vi "Spectrogram demo.vi"() -> ()   [LabVIEW 2018]
uses:
  <vilib>/Analysis/NI_AALBase.lvlib
  <vilib>/gmath/NI_Gmath.lvlib
  <vilib>/Analysis/NI_AALPro.lvlib
panel:
  in  "Stop":bool
  out "STFT Spectrogram":dbl[][](graph)
  in  "Signal":u16(ring) items=["Chirp", "Sine ", "Heart Sound ", "Arbitrary"]
  in  "Arbitrary Formula":string="sin(1000*t)*exp(t*t)*sin(500*t*t)*(exp(t))"
  out "OK":bool
  in  "Map selector":T1(ring)=enum."rainbow"
  out "Acquired time domain signal":waveform(dbl)(graph)={"t0"=timestamp(0 s since 1904-01-01), "dt"=0.001, "Y"=[]}
  in  "Window parameter":dbl=nan
  in  "Type":u32(ring)=1 items=["Rectangle"=0, "Hanning"=1, "Hamming"=2, "Blackman-Harris"=3, "Exact Blackman"=4, "Blackman"=5, "Flat Top"=6, "4 Term B-Harris "=7, "7 Term B-Harris"=8, "Low Sidelobe"=9, "Blackman Nuttall"=11, "Triangle"=30, "Bartlett-Hanning"=31, "Bohman"=32, "Parzen"=33, "Welch"=34, "Kaiser"=60, "Dolph-Chebyshev"=61, "Gaussian"=62]
  in  "Length":i32=64
  out "Power Spectrum":cluster{"Power Spectrum (V^2 rms)":dbl[], dbl[]}(graph)
  in  "Time steps":i32(slide)=2 scale=2.0..20.0
  in  "Frequency bins":i32=512
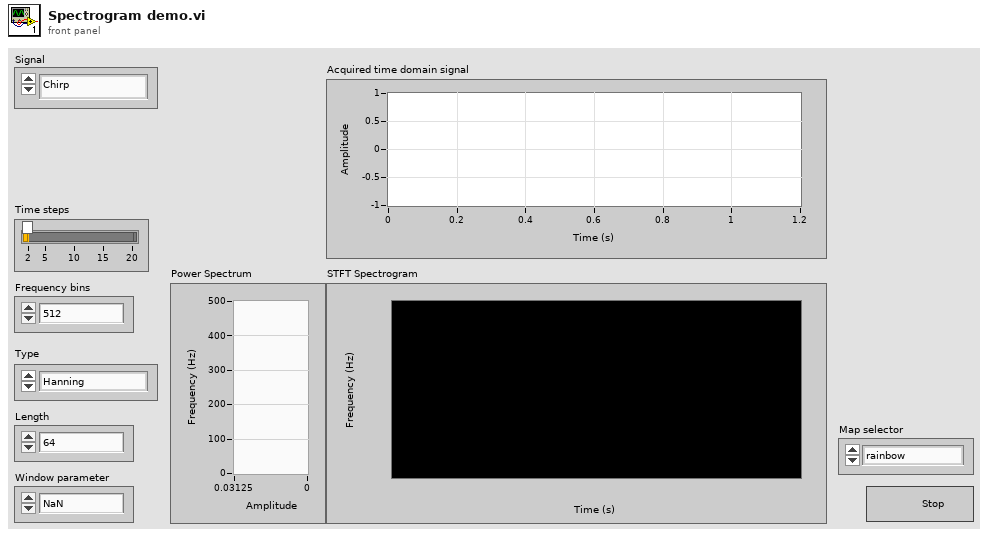
[diagram p1: front panel]
types:
  T1 = enum16{"fire", "rainbow", "grey", "inverse grey", "ice", "original"}
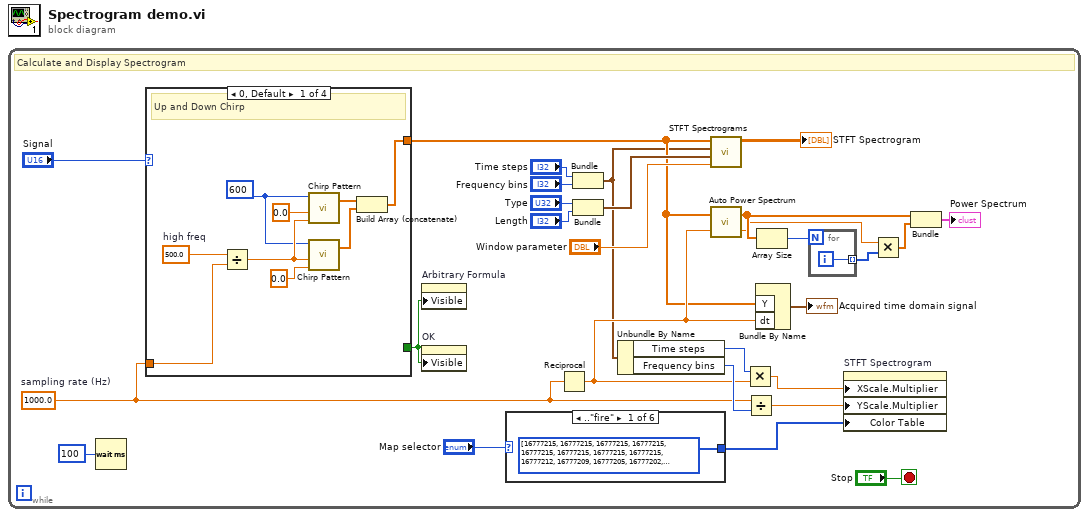
[diagram p0: block diagram]
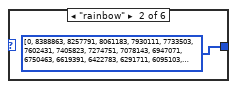
[diagram p2: hidden frame]
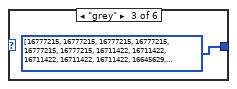
[diagram p3: hidden frame]
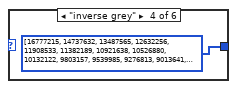
[diagram p4: hidden frame]
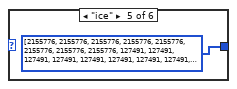
[diagram p5: hidden frame]
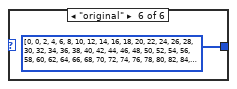
[diagram p6: hidden frame]
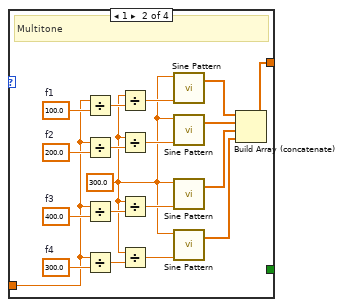
[diagram p7: hidden frame]
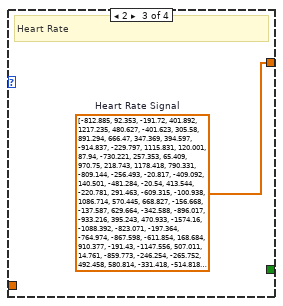
[diagram p8: hidden frame]
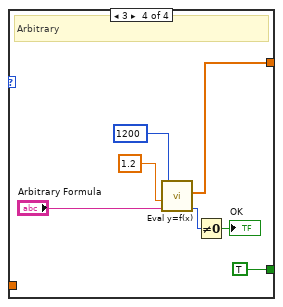
[diagram p9: hidden frame]
diagram:
  n1 = while {
    stop <- "Stop" stop-if-true
    w13 = 1000.0  # sampling rate (Hz)
    # "Calculate and Display Spectrogram"
    n2 = Wait (ms)(milliseconds to wait=u32 100 ("millisecond multiple")) -> ()  [unwired: 1 out]
    n3 = case shown="0, Default" "Signal" {
      tunnel: [w40 w46 w64 w65] -> w10
      tunnel: w13 -> [w39 w45 _ _]
      tunnel: [_ _ _ TRUE ("Visible")] -> w8
      frame 0, Default {
        w38 = 500.0  # high freq
        w36 = 600 ("samples")
        # "Up and Down Chirp"
        n4 = Divide(x=w38, y=w39) -> (x/y=w37:dbl)
        n5 = call <vilib>:"Chirp Pattern.vi"("f2"=w37, "f1"=0.0, "samples"=w36) -> ("Chirp Pattern"=w43:dbl[])  [unwired: 1 in, 1 out]
        n6 = call <vilib>:"Chirp Pattern.vi"("f2"=0.0, "f1"=w37, "samples"=w36) -> ("Chirp Pattern"=w44:dbl[])  [unwired: 1 in, 1 out]
        n7 = Build Array (concatenate)(w43, w44) -> (w40:dbl[])
      }
      frame 1 {
        w53 = 300.0  # f4
        w56 = 400.0  # f3
        w60 = 200.0  # f2
        w63 = 100.0  # f1
        w51 = 300.0 ("samples")
        # "Multitone"
        n8 = Divide(x=w45, y=w63) -> (x/y=w62:dbl)
        n9 = Divide(x=w45, y=w60) -> (x/y=w59:dbl)
        n10 = Divide(x=w45, y=w56) -> (x/y=w57:dbl)
        n11 = Divide(x=w45, y=w53) -> (x/y=w52:dbl)
        n12 = Divide(x=w51, y=w62) -> (x/y=w61:dbl)
        n13 = Divide(x=w51, y=w59) -> (x/y=w58:dbl)
        n14 = Divide(x=w51, y=w57) -> (x/y=w55:dbl)
        n15 = Divide(x=w51, y=w52) -> (x/y=w54:dbl)
        n16 = call <vilib>:"Sine Pattern.vi"("cycles"=w61, "samples"=w51) -> ("Sinusoidal Pattern"=w50:dbl[])  [unwired: 2 in, 1 out]
        n17 = call <vilib>:"Sine Pattern.vi"("cycles"=w58, "samples"=w51) -> ("Sinusoidal Pattern"=w49:dbl[])  [unwired: 2 in, 1 out]
        n18 = call <vilib>:"Sine Pattern.vi"("cycles"=w55, "samples"=w51) -> ("Sinusoidal Pattern"=w48:dbl[])  [unwired: 2 in, 1 out]
        n19 = call <vilib>:"Sine Pattern.vi"("cycles"=w54, "samples"=w51) -> ("Sinusoidal Pattern"=w47:dbl[])  [unwired: 2 in, 1 out]
        n20 = Build Array (concatenate)(w50, w49, w48, w47) -> (w46:dbl[])
      }
      frame 2 {
        w64 = dbl[] [-812.885, 92.353, -191.72, 401.892, 1217.235, 480.627, -401.623, 305.58, 891.294, 666.47, 347.369, 394.597, -914.837, -229.797, 1115.831, 120.001, 87.94, -730.221, 257.353, 65.409, 970.75, 218.743, 1178.418, 790.331, -809.144, -256.493, -20.817, -409.092, 140.501, -481.284, -20.54, 413.544, -220.781, 291.463, -609.315, -100.938, 1086.714, 570.445, 668.827, -156.668, -137.587, 629.664, -342.588, -896.017, -933.216, 395.243, 470.933, -1574.16, -1088.392, -823.071, -197.364, -764.974, -867.598, -611.854, 168.684, 910.377, -191.43, -1147.556, 507.011, 14.761, -859.773, -246.254, -265.752, 492.458, 580.814, -331.418, -514.818, -447.725, 454.298, 888.117, 582.526, -181.283, 133.12, 455.725, 220.22, 171.147, -399.537, 589.594, 576.944, 612.789, -284.778, 129.553, 280.847, -908.959, 154.83, -223.049, -792.168, -628.228, -114.823, -737.632, 401.997, -149.505, 384.074, -223.453, 543.075, 234.777, -510.364, 515.33, 1229.174, -76.426, 79.706, -372.049, -119.862, -159.57, 644.837, 95.055, 161.962, 119.439, 512.005, 457.789, 502.756, -572.27, -363.025, -861.699, -690.604, -306.68, -280.622, 354.958, 718.783, -635.96, -661.983, -1036.168, 933.818, -21.857, 481.32, -595.728, 413.466, -546.083, 22.21, 647.591, -532.26, -6.045, -598.047, -1127.544, 339.862, 71.452, 1404.022, 664.043, 187.514, -674.093, 727.214, 380.689, 809.771, 189.41, 270.586, -308.498, -275.665, -976.634, -36.294, 65.959, -456.042, 376.845, -767.07, -834.083, 166.988, -761.587, 1313.221, 549.851, -141.967, -478.882, 332.027, -197.81, 243.895, 178.342, -1065.602, 370.738, 737.347, -638.379, 273.486, 147.083, 507.727, 366.731, -172.42, 82.989, 275.166, -395.509, 141.831, 345.849, 492.327, 164.523, -306.638, 48.493, 1131.402, -269.039, -223.141, 653.685, 345.058, -556.369, 183.304, 167.256, -515.512, -1185.376, -715.82, 1379.127, 76.647, -444.987, 484.532, -400.697, 134.075, 307.371, -573.019, 798.681, 851.811, -227.385, -184.374, 398.144, -624.698, 1077.018, 396.243, 505.665, 215.136, 667.812, 850.606, 458.682, 75.092, 415.742, 796.084, 613.509, -120.458, 331.781, 645.796, -6.721, 450.739, -676.773, -494.105, -479.193, 540.918, 866.113, 525.902, -163.718, 15.87, -335.594, -751.403, 364.11, 856.606, 1452.089, 1002.265, -532.028, -3042.086, -2031.079, -373.696, 3030.349, 4520.987, 1649.755, -3455.973, -8843.97, -6968.636, 2697.603, 11653.749, 9076.124, -505.548, -10855.807, -11188.486, -1440.078, 10736.562, 11563.332, 2957.903, -8571.92, -9999.609, -4041.165, 5183.188, 7578.477, 1954.224, -2758.964, -4444.383, -1189.552, 1155.772, 2622.929, 1181.467, -1496.027, -956.537, 804.996, -1017.112, 509.03, 111.684, -447.935, -367.205, -293.243, -827.365, -64.065, -420.348, -575.659, 333.719, 366.484, -332.705, 1380.656, 564.165, 478.851, 820.87, 595.132, 902.574, -277.885, 565.918, -41.599, 162.17, -196.852, 474.902, -646.552, 1162.594, 239.658, 412.565, -228.316, 479.864, 176.821, -1645.903, -1043.217, -313.404, -641.977, -670.528, 12.622, -732.982, -820.426, 679.662, 163.281, -173.538, 203.833, -264.991, 699.957, 131.238, 104.042, -266.732, 119.745, -187.847, -423.473, 214.622, 361.945, -120.424, 628.229, 103.454, 416.288, 447.196, 1998.638, 459.144, -507.876, -510.127, 444.898, 286.278, 141.479, 856.694, 704.954, -481.379, 199.402, 402.743, 763.071, 477.005, -238.528, 175.67, -1070.44, -210.356, -563.045, -254.9, -269.013, 242.621, -122.229, 1244.566, -1511.321, 770.062, -123.879, -315.28, 161.941, -369.078, -650.285, 154.461, 668.199, -536.558, -636.982, 827.007, 563.321, 307.414, 416.868, -813.524, 187.769, -47.802, -377.969, 134.803, 479.919, 104.555, 76.347, 122.435, 461.959, 712.356, 855.744, 643.533, -299.323, 29.123, -611.322, -243.59, -57.464, -241.028, 292.484, -530.522, -953.832, 213.495, 1019.907, -146.036, -451.208, -316.589, -483.618, 1040.822, 582.644, -930.517, 1047.99, 386.527, -790.048, -289.878, -319.321, -758.195, -39.781, -135.797, 941.554, 473.63, 314.691, 962.971, 293.801, 357.646, -79.738, 1228.183, 666.349, -1313.84, 253.291, 2280.083, -2911.26, -2377.851, 3105.478, 3919.796, -4843.257, -6974.238, 4525.842, 9923.63, -3291.479, -12103.127, -4759.899, 12469.517, 10124.81, -6179.313, -15608.631, -5502.488, 10177.794, 13405.504, 1557.947, -10712.939, -11430.111, -609.233, 9526.937, 7951.213, 1792.035, -4464.963, -6766.333, -4418.031, -667.07, 2860.936, 2093.854, 1731.777, -818.7, -1113.903, -987.711, -1048.25, -471.31, 794.256, 326.182, -592.837, 426.692, 669.155, -551.359, -1330.657, -744.817, 291.008, 940.554, -575.586, 120.746, -201.647, -181.902, -577.326, -153.09, -147.901, 852.486, -150.707, 165.594, 388.62, -500.968, 830.494, -196.448, -722.129, 1701.033, 805.591, -688.984, 480.594, -442.062, -1157.85, -331.575, -847.915, -749.434, -280.289, -48.062, -321.303, -175.183, 390.326, -295.451, 860.076, 4.215, -291.954, 1194.712, 107.477, 775.875, -569.583, 658.765, -757.795, -220.891, 232.347, 135.744, 27.832, -128.671, -861.785, -109.875, -417.782, -831.565, -336.154, -237.548, -289.505, 3.085, 546.202, -427.676, 298.979, -1146.466, -30.704, -91.479, 801.289, -444.648, -5.801, 734.655, -575.291, -108.679, 15.505, -162.351, 754.145, 324.503, -464.294, 1065.479, 164.281, 811.698, -95.714, -459.461, 137.022, 230.538, 62.256, -363.207, 399.628, -107.244, 720.175, 1489.831, 432.423, -352.224, -1389.143, 1218.703, -156.439, 617.235, 763.837, -3.486, -813.677, -219.988, 694.033, -613.495, -262.113, -725.543, 538.351, -974.242, -641.106, -623.892, -151.01, -4.086, -1029.322, 300.303, 80.614, 36.968, -450.02, -882.371, 538.339, -266.879, 950.849, 192.847, -30.885, 216.172, 49.234, -707.738, -1028.599, -356.354, -767.614, 588.727, 92.207, 59.365, 193.588, 418.274, 157.459, 1060.452, -708.044, 390.038, 106.017, 132.994, 429.056, -523.781, -964.161, 85.288, -214.823, 166.293, -847.485, 594.838, 137.015, 143.776, 515.996, 779.295, 971.556, 552.461, 206.866, 910.451, -771.806, 19.76, 265.241, 641.013, -500.539, 592.25, 1138.402, -1019.78, -132.543, 671.621, -275.528, 339.8, -710.534, -527.259, -680.392, -823.823, -475.58, -1319.165, 665.25, 859.226, -122.816, 449.975, -608.928, 757.932, -1141.948, -347.354, 1101.294, 542.32, 257.838, 107.018, 471.874, -675.938, 210.467, 488.136, 369.739, 494.873, -304.293, 362.761, -198.079, -678.376, 196.02, 1567.826, -411.872, 635.674, 614.003, 447.948, -575.023, 24.269, 138.156, 990.358, 23.976, 212.611, 506.072, 809.328, 86.246, -158.537, -948.734, 418.084, 529.828, -573.065, -544.773, -559.736, -293.086, 145.955, 564.455, 284.711, -267.396, -470.639, 66.951, -305.952, 1079.132, 119.481, 183.056, -218.108, 220.327, 956.435, 879.341, 142.07, 285.57, 182.042, 499.017, -414.272, 618.006, -110.562, 363.038, 1226.001, -13.947, 317.896, 332.134, -427.275, -324.199, 165.785, -148.066, 832.505, 545.739, 572.835, -698.079, -796.558, 876.564, 1035.197, -502.461, 88.961, -125.865, 435.317, 573.484, -693.412, -820.951, -221.263, 34.476, 350.548, -814.032, 1302.716, 292.15, -206.114, -990.355, -528.934, 2.093, 753.912, -170.46, -860.099, 314.44, -706.064, -82.74, -961.794, 911.057, 1190.978, -758.438, -317.119, -370.116, 344.094, 2.734, -411.061, 153.438, -29.571, 61.242, -206.535, -145.31, 540.441, -583.685, -69.607, -514.175, 178.811, -510.477, -382.528, -866.248, -10.829, -1206.153, 42.783, 387.505, -1191.419, 607.521, 58.531, -424.03, -325.545, 490.254, 226.705, 404.271, 365.632, -659.777, -172.052, -412.707, 860.262, -1013.23, 386.705, 91.511, -1137.016, -250.362, 81.086, -459.153, -312.97, -964.309, 807.672, -446.647, -761.347, 22.545, -755.565, 1344.585, -552.501, 135.409, -440.169, -263.736, 546.636, 937.931, -787.274, -75.41, 687.59, -18.132, 1218.893, 1385.113, 660.538, -513.578, -328.177, -2484.127, -2621.497, -509.223, 6386.645, 9015.466, 5036.201, -6680.306, -14787.188, -8640.573, 7594.916, 14338.31, 2948.091, -9228.146, -6642.571, 2936.511, 5094.057, 126.975, -2716.489, -902.238, 727.639, 840.681, 377.892, -1398.395, 324.266, 1320.751, -211.398, -915.179, -789.013, -597.323, 537.766, -239.827, -482.099, -909.184, 1249.653, -39.083, 529.925, 41.638, 161.626, 836.279, 154.883, -751.712, 43.625, -534.923, 65.24, -119.906, -2.542, 1701.32, -875.16, 797.924, -855.379, -339.916, 773.776, 578.232, 55.307, -105.059, -392.251, 525.32, -676.284, -913.689, 118.783, -157.711, -107.748, -805.284, -125.231, 531.254, -1005.267, -152.386, -185.309, 151.891, 549.237, 1460.491, 718.276, -703.941, 443.496, 44.347, -575.276, 227.804, -318.171, 286.076, -52.271, -158.905, 47.149, 732.895, 818.402, -175.499, -476.743, 102.837, 484.994, 375.355, 286.881, -321.417, 83.485, -591.817, 668.815, -1135.234, -632.803, -163.511, -68.345, 175.9, 1045.329, -214.271, 202.611, 790.612, 148.964, -495.302, -228.243, 1358.566, -1346.808, 173.046, 318.1, 647.317, 140.127, -280.934, 265.519, 222.671, -307.83, 160.312, 718.053, 531.692, 645.59, 371.401, 49.052, -318.111, -268.433, -179.362, 52.268, -301.64, -358.636, 877.188, 931.345, -1239.939, -1066.649, 963.904, -1510.834, -333.052, 115.87, 119.453, 300.372, 110.794, -431.006, 56.819, 661.49, 39.005, -160.524, 813.758, 343.281, 1339.01, 306.876, 468.435, -645.293, -307.609, -1822.453, -12.383, -102.888, -280.243, -788.583, 148.947, 115.909, -559.586, -655.272, -639.815, -590.54, 66.557, 289.129, 11.823, -62.432, 330.158, 281.538, -1039.723, 361.93, 474.581, 1068.964, -298.894, 170.574, -438.046, 349.506, 1506.718, 605.084, -1480.066, -2709.404, -262.503, 4480.743, 2691.419, -2281.395, -8278.374, -3183.168, 8229.434, 11058.8, -340.125, -13611.163, -11549.902, 1960.208, 13751.73, 10465.135, -2599.744, -12490.653, -8526.591, 2779.39, 8025.551, 4521.424, -1594.693, -3575.465, -3622.377, 138.034, 1818.082, 1236.288, -317.301, 14.132, -112.302, -819.945, 49.762, -788.421, -339.472, 1531.908, -119.728, 729.993, 149.62, -121.858, 536.013, -92.935, 416.223, 181.051, -125.007, -129.572, 44.364, -349.327, -176.383, -377.563, 961.207, -458.841, -412.175, -634.75, 10.515, 264.715, -881.101, 750.742, 468.51, -1085.815, 150.164, -379.086, -1561.12, 201.207, -1086.201, 613.288, 78.072, 1171.668, 756.135, 492.25, 426.936, 992.188, 882.106, 42.81, -265.932, 110.589, -28.026, -747.429, 329.531, -71.608, 943.605, -362.701, -253.425, 297.224, -1183.985, 176.766, 426.989, -1067.177, 120.913, -42.309, 825.667, 939.997, 461.771, -447.707, -890.955, -778.78, -393.755, 1006.719, -1175.487, 214.889, -788.833, 579.234, 1078.956, -19.185, -282.586, -101.411, 192.631, 533.567, -423.696, 316.108, 1526.409, 727.392, 441.79, 854.429, -119.848, -406.14, -478.996, -927.949, -614.602, -57.838, 331.653, -561.592, 327.492, -152.725, -156.28, 740.983, -11.85, 539.567, -67.788, 73.723, 149.398, 1012.716, 906.524, 841.835, 182.924, 62.797, -147.373, -767.301, 515.692, 1046.049, -271.503, 993.61, 748.723, 340.694, 473.367, -170.699, 562.102, 517.643, 502.045, 421.43, -659.886, -247.582, 265.233, -621.61, 440.326, 80.707, 359.761, -527.815, -59.844, -690.419, 1572.515, 489.455, -50.783, -272.113, -33.808, 865.43, 810.077, -29.446, 1204.538, 18.474, 328.274, 881.365, 375.371, 871.262, -307.907, -35.284, -450.565, -368.036, 505.55, 3.446, 161.214, -261.762, 519.098, -150.873, -18.037, 465.692, -601.507, -327.262, -244.804, 317.025, 77.043, -380.644, -771.317, 224.907, -234.73, 135.903, 413.949, -289.456, -20.991, 169.481, 363.244, 466.716, 1.778, -376.402, 342.312, 257.517, -144.621, 611.87, 1171.643, -79.737, -621.343, 219.535, -399.15, 203.735, -624.161, 168.41]  # Heart Rate Signal
        # "Heart Rate"
      }
      frame 3 {
        # "Arbitrary"
        n21 = call <vilib>:"Eval y=f(x).vi"("formula"="Arbitrary Formula", "end"=1.2, "number of points"=u32 1200) -> ("error"=w67:i32, "Y Values"=w65:dbl[])  [unwired: 1 in, 2 out]
        n22 = Not Equal To 0?(x=w67) -> (x != 0?=→"OK":bool)
      }
    }
    n23 = property on="Arbitrary Formula" class="Str"("Visible"=w8) -> ()  [unwired: 2 in, 2 out]
    n24 = property on="OK" class="Bool"("Visible"=w8) -> ()  [unwired: 2 in, 2 out]
    n25 = case shown="..\"fire\"" "Map selector" {
      tunnel: [u32[] [16777215, 16777215, 16777215, 16777215, 16777215, 16777215, 16777215, 16777215, 16777212, 16777209, 16777205, 16777202, 16777199, 16777196, 16777193, 16777190, 16777186, 16777183, 16777180, 16777177, 16777174, 16777170, 16777167, 16777164, 16777161, 16777158, 16777154, 16777151, 16777148, 16777145, 16777142, 16777139, 16777135, 16777132, 16777129, 16777126, 16777123, 16777119, 16777116, 16777113, 16777110, 16777107, 16777103, 16777100, 16777097, 16777094, 16777091, 16777088, 16777084, 16777081, 16777078, 16777075, 16777072, 16777068, 16777065, 16777062, 16777059, 16777056, 16777052, 16777049, 16777046, 16777043, 16777040, 16777037, 16777033, 16777030, 16777027, 16777024, 16777021, 16777017, 16777014, 16777011, 16777008, 16777005, 16777001, 16776998, 16776995, 16776992, 16776989, 16776986, 16776982, 16776979, 16776976, 16776973, 16776970, 16776966, 16776963, 16776960, 16776192, 16775424, 16774400, 16773632, 16772864, 16772096, 16771328, 16770560, 16769536, 16768768, 16768000, 16767232, 16766464, 16765440, 16764672, 16763904, 16763136, 16762368, 16761344, 16760576, 16759808, 16759040, 16758272, 16757504, 16756480, 16755712, 16754944, 16754176, 16753408, 16752384, 16751616, 16750848, 16750080, 16749312, 16748288, 16747520, 16746752, 16745984, 16745216, 16744448, 16743424, 16742656, 16741888, 16741120, 16740352, 16739328, 16738560, 16737792, 16737024, 16736256, 16735232, 16734464, 16733696, 16732928, 16732160, 16731392, 16730368, 16729600, 16728832, 16728064, 16727296, 16726272, 16725504, 16724736, 16723968, 16723200, 16722176, 16721408, 16720640, 16719872, 16719104, 16718336, 16717312, 16716544, 16715776, 16715008, 16714240, 16713216, 16712448, 16711680, 16515072, 16318464, 16056320, 15859712, 15663104, 15466496, 15269888, 15073280, 14811136, 14614528, 14417920, 14221312, 14024704, 13762560, 13565952, 13369344, 13172736, 12976128, 12713984, 12517376, 12320768, 12124160, 11927552, 11730944, 11468800, 11272192, 11075584, 10878976, 10682368, 10420224, 10223616, 10027008, 9830400, 9633792, 9371648, 9175040, 8978432, 8781824, 8585216, 8388608, 8126464, 7929856, 7733248, 7536640, 7340032, 7077888, 6881280, 6684672, 6488064, 6291456, 6029312, 5832704, 5636096, 5439488, 5242880, 5046272, 4784128, 4587520, 4390912, 4194304, 3997696, 3735552, 3538944, 3342336, 3145728, 2949120, 2686976, 2490368, 2293760, 2097152, 1900544, 1703936, 1441792, 1245184, 1048576, 851968, 655360, 393216, 196608, 65793, 65793, 65793, 65793, 65793, 65793, 65793, 65793, 0] ("256 fire") u32[] [0, 8388863, 8257791, 8061183, 7930111, 7733503, 7602431, 7405823, 7274751, 7078143, 6947071, 6750463, 6619391, 6422783, 6291711, 6095103, 5964031, 5767423, 5636351, 5439743, 5308671, 5112063, 4980991, 4784383, 4653311, 4456703, 4325631, 4129023, 3932415, 3801343, 3604735, 3473663, 3277055, 3145983, 2949375, 2818303, 2621695, 2490623, 2294015, 2162943, 1966335, 1835263, 1638655, 1507583, 1310975, 1179903, 983295, 852223, 655615, 524543, 327935, 196863, 511, 1791, 3071, 4351, 5631, 6911, 8191, 9471, 10751, 12031, 13311, 14591, 15871, 17151, 18431, 19711, 20991, 22271, 23551, 24831, 26111, 27391, 28671, 29951, 31231, 32511, 33791, 35071, 36351, 37631, 38911, 40191, 41471, 42751, 44031, 45311, 46591, 47871, 49151, 50431, 51711, 52991, 54271, 55551, 56831, 58111, 59391, 60671, 61951, 63231, 64511, 65532, 65527, 65522, 65517, 65512, 65507, 65502, 65497, 65492, 65487, 65482, 65477, 65472, 65467, 65462, 65457, 65452, 65447, 65442, 65437, 65432, 65427, 65422, 65417, 65412, 65407, 65402, 65397, 65392, 65387, 65382, 65377, 65372, 65367, 65362, 65357, 65352, 65347, 65342, 65337, 65332, 65327, 65322, 65317, 65312, 65307, 65302, 65297, 65292, 65287, 65282, 261888, 589568, 917248, 1244928, 1572608, 1900288, 2227968, 2555648, 2883328, 3211008, 3538688, 3866368, 4194048, 4521728, 4849408, 5177088, 5504768, 5832448, 6160128, 6487808, 6815488, 7143168, 7470848, 7798528, 8126208, 8453888, 8781568, 9109248, 9436928, 9764608, 10092288, 10419968, 10747648, 11075328, 11403008, 11730688, 12058368, 12386048, 12713728, 13041408, 13369088, 13696768, 14024448, 14352128, 14679808, 15007488, 15335168, 15662848, 15990528, 16318208, 16645888, 16775936, 16774656, 16773376, 16772096, 16770816, 16769536, 16768256, 16766976, 16765696, 16764416, 16763136, 16761856, 16760576, 16759296, 16758016, 16756736, 16755456, 16754176, 16752896, 16751616, 16750336, 16749056, 16747776, 16746496, 16745216, 16743936, 16742656, 16741376, 16740096, 16738816, 16737536, 16736256, 16734976, 16733696, 16732416, 16731136, 16729856, 16728576, 16727296, 16726016, 16724736, 16723456, 16722176, 16720896, 16719616, 16718336, 16717056, 16715776, 16714496, 16713216, 16711680] ("rainbow") u32[] [16777215, 16777215, 16777215, 16777215, 16777215, 16777215, 16711422, 16711422, 16711422, 16711422, 16711422, 16645629, 16645629, 16645629, 16645629, 16645629, 16645629, 16579836, 16579836, 16579836, 16579836, 16579836, 16514043, 16514043, 16514043, 16514043, 16514043, 16448250, 16448250, 16448250, 16448250, 16448250, 16316664, 16382457, 16382457, 16382457, 16382457, 16316664, 16316664, 16316664, 16316664, 16250871, 16250871, 16250871, 16250871, 16250871, 16185078, 16185078, 16185078, 16185078, 16119285, 16119285, 16119285, 16119285, 16119285, 16053492, 16053492, 16053492, 16053492, 15987699, 15987699, 15987699, 15987699, 15921906, 15987699, 15921906, 15921906, 15856113, 15856113, 15856113, 15856113, 15856113, 15790320, 15790320, 15790320, 15724527, 15724527, 15724527, 15724527, 15658734, 15658734, 15658734, 15658734, 15592941, 15592941, 15592941, 15592941, 15527148, 15527148, 15527148, 15461355, 15461355, 15461355, 15461355, 15395562, 15395562, 15395562, 15395562, 15329769, 15329769, 15329769, 15263976, 15263976, 15263976, 15198183, 15198183, 15198183, 15198183, 15132390, 15132390, 15132390, 15066597, 15066597, 15066597, 15000804, 15000804, 15000804, 14935011, 14935011, 14935011, 14869218, 14869218, 14869218, 14803425, 14803425, 14803425, 14737632, 14737632, 14671839, 14671839, 14671839, 14606046, 14606046, 14606046, 14540253, 14540253, 14540253, 14474460, 14474460, 14408667, 14408667, 14408667, 14342874, 14342874, 14277081, 14277081, 14277081, 14211288, 14211288, 14145495, 14145495, 14079702, 14079702, 14013909, 14013909, 14013909, 13948116, 13948116, 13882323, 13882323, 13816530, 13816530, 13750737, 13750737, 13684944, 13684944, 13619151, 13619151, 13553358, 13553358, 13487565, 13487565, 13421772, 13421772, 13355979, 13290186, 13290186, 13224393, 13224393, 13158600, 13092807, 13092807, 13027014, 13027014, 12961221, 12895428, 12895428, 12829635, 12763842, 12763842, 12698049, 12632256, 12566463, 12566463, 12500670, 12434877, 12434877, 12369084, 12303291, 12237498, 12171705, 12171705, 12105912, 12040119, 11974326, 11908533, 11842740, 11776947, 11711154, 11645361, 11579568, 11513775, 11447982, 11382189, 11316396, 11250603, 11184810, 11119017, 10987431, 10921638, 10855845, 10790052, 10658466, 10592673, 10461087, 10395294, 10329501, 10197915, 10066329, 10000536, 9868950, 9737364, 9605778, 9474192, 9342606, 9211020, 9079434, 8882055, 8750469, 8553090, 8421504, 8224125, 7960953, 7763574, 7500402, 7237230, 6974058, 6645093, 6316128, 5855577, 5395026, 4868682, 4210752, 3289650, 2105376, 0] ("256 log up") u32[] [16777215, 14737632, 13487565, 12632256, 11908533, 11382189, 10921638, 10526880, 10132122, 9803157, 9539985, 9276813, 9013641, 8816262, 8553090, 8421504, 8224125, 8026746, 7895160, 7697781, 7566195, 7434609, 7303023, 7171437, 7039851, 6908265, 6776679, 6710886, 6579300, 6447714, 6381921, 6316128, 6184542, 6118749, 5987163, 5921370, 5855577, 5789784, 5658198, 5592405, 5526612, 5460819, 5395026, 5329233, 5263440, 5197647, 5131854, 5066061, 5000268, 4934475, 4868682, 4802889, 4737096, 4671303, 4605510, 4605510, 4539717, 4473924, 4408131, 4342338, 4342338, 4276545, 4210752, 4210752, 4144959, 4079166, 4013373, 4013373, 3947580, 3881787, 3881787, 3815994, 3750201, 3750201, 3684408, 3684408, 3618615, 3552822, 3552822, 3487029, 3487029, 3421236, 3421236, 3355443, 3289650, 3289650, 3223857, 3223857, 3158064, 3158064, 3092271, 3092271, 3026478, 3026478, 2960685, 2960685, 2894892, 2894892, 2829099, 2829099, 2763306, 2763306, 2763306, 2697513, 2697513, 2631720, 2631720, 2565927, 2565927, 2500134, 2500134, 2500134, 2434341, 2434341, 2368548, 2368548, 2368548, 2302755, 2302755, 2236962, 2236962, 2236962, 2171169, 2171169, 2171169, 2105376, 2105376, 2105376, 2039583, 2039583, 1973790, 1973790, 1973790, 1907997, 1907997, 1907997, 1842204, 1842204, 1842204, 1776411, 1776411, 1776411, 1710618, 1710618, 1710618, 1644825, 1644825, 1644825, 1579032, 1579032, 1579032, 1579032, 1513239, 1513239, 1513239, 1447446, 1447446, 1447446, 1381653, 1381653, 1381653, 1381653, 1315860, 1315860, 1315860, 1315860, 1250067, 1250067, 1250067, 1184274, 1184274, 1184274, 1184274, 1118481, 1118481, 1118481, 1118481, 1052688, 1052688, 1052688, 1052688, 986895, 986895, 986895, 921102, 921102, 921102, 921102, 921102, 855309, 855309, 855309, 855309, 789516, 789516, 789516, 789516, 723723, 723723, 723723, 723723, 657930, 657930, 657930, 657930, 657930, 592137, 592137, 592137, 592137, 526344, 526344, 526344, 526344, 526344, 460551, 460551, 460551, 460551, 460551, 394758, 394758, 394758, 394758, 328965, 328965, 328965, 328965, 328965, 263172, 263172, 263172, 263172, 263172, 197379, 197379, 197379, 197379, 197379, 131586, 131586, 131586, 131586, 131586, 131586, 65793, 65793, 65793, 65793, 65793, 0, 0, 0, 0, 0, 0] ("256 log down") u32[] [2155776, 2155776, 2155776, 2155776, 2155776, 2155776, 2155776, 2155776, 127491, 127491, 127491, 127491, 127491, 127491, 127491, 127491, 522752, 522752, 522752, 522752, 522752, 522752, 522752, 522752, 64018, 64018, 64018, 64018, 64018, 64018, 64018, 64018, 63778, 63778, 63778, 63778, 63778, 63778, 63778, 63778, 63790, 63790, 63790, 63790, 63790, 63790, 63790, 63790, 63797, 63797, 63797, 63797, 63797, 63797, 63797, 63797, 63807, 63807, 63807, 63807, 63807, 63807, 63807, 63807, 64068, 64068, 64068, 64068, 64068, 64068, 64068, 64068, 63828, 63828, 63828, 63828, 63828, 63828, 63828, 63828, 63833, 63833, 63833, 63833, 63833, 63833, 63833, 63833, 63836, 63836, 63836, 63836, 63836, 63836, 63836, 63836, 63836, 63836, 63836, 63836, 63836, 63836, 63836, 63836, 61790, 61790, 61790, 61790, 61790, 61790, 61790, 61790, 58464, 58464, 58464, 58464, 58464, 58464, 58464, 58464, 55387, 55387, 55387, 55387, 55387, 55387, 55387, 55387, 51286, 51286, 51286, 51286, 51286, 51286, 51286, 51286, 47440, 47440, 47440, 47440, 47440, 47440, 47440, 47440, 40284, 40284, 40284, 40284, 40284, 40284, 40284, 40284, 34154, 34154, 34154, 34154, 34154, 34154, 34154, 34154, 28540, 28540, 28540, 28540, 28540, 28540, 28540, 28540, 20113, 20113, 20113, 20113, 20113, 20113, 20113, 20113, 12193, 12193, 12193, 12193, 12193, 12193, 12193, 12193, 12714, 12714, 12714, 12714, 12714, 12714, 12714, 12714, 7351, 7351, 7351, 7351, 7351, 7351, 7351, 7351, 4800, 4800, 4800, 4800, 4800, 4800, 4800, 4800, 195, 195, 195, 195, 195, 195, 195, 195, 189, 189, 189, 189, 189, 189, 189, 189, 183, 183, 183, 183, 183, 183, 183, 183, 175, 175, 175, 175, 175, 175, 175, 175, 164, 164, 164, 164, 164, 164, 164, 164, 155, 155, 155, 155, 155, 155, 155, 155] ("32 ice") u32[] [0, 0, 2, 4, 6, 8, 10, 12, 14, 16, 18, 20, 22, 24, 26, 28, 30, 32, 34, 36, 38, 40, 42, 44, 46, 48, 50, 52, 54, 56, 58, 60, 62, 64, 66, 68, 70, 72, 74, 76, 78, 80, 82, 84, 86, 88, 90, 92, 94, 96, 98, 100, 102, 104, 106, 108, 110, 112, 114, 116, 118, 120, 122, 124, 126, 128, 130, 132, 134, 136, 138, 140, 142, 144, 146, 148, 150, 152, 154, 156, 158, 160, 162, 164, 166, 168, 170, 172, 174, 176, 178, 180, 182, 184, 186, 188, 190, 192, 194, 196, 198, 200, 202, 204, 206, 208, 210, 212, 214, 216, 218, 220, 222, 224, 226, 228, 230, 232, 234, 236, 238, 240, 242, 244, 246, 248, 250, 252, 255, 131839, 263423, 395007, 526591, 658175, 789759, 921343, 1052927, 1184511, 1316095, 1447679, 1579263, 1710847, 1842431, 1974015, 2105599, 2237183, 2368767, 2500351, 2631935, 2763519, 2895103, 3026687, 3158271, 3289855, 3421439, 3553023, 3684607, 3816191, 3947775, 4079359, 4210943, 4342527, 4474111, 4605695, 4737279, 4868863, 5000447, 5132031, 5263615, 5395199, 5526783, 5658367, 5789951, 5921535, 6053119, 6184703, 6316287, 6447871, 6579455, 6711039, 6842623, 6974207, 7105791, 7237375, 7368959, 7500543, 7632127, 7763711, 7895295, 8026879, 8158463, 8290047, 8421631, 8553215, 8684799, 8816383, 8947967, 9079551, 9211135, 9342719, 9474303, 9605887, 9737471, 9869055, 10000639, 10132223, 10263807, 10395391, 10526975, 10658559, 10790143, 10921727, 11053311, 11184895, 11316479, 11448063, 11579647, 11711231, 11842815, 11974399, 12105983, 12237567, 12369151, 12500735, 12632319, 12763903, 12895487, 13027071, 13158655, 13290239, 13421823, 13553407, 13684991, 13816575, 13948159, 14079743, 14211327, 14342911, 14474495, 14606079, 14737663, 14869247, 15000831, 15132415, 15263999, 15395583, 15527167, 15658751, 15790335, 15921919, 16053503, 16185087, 16316671, 16448255, 16579839, 16777215] ("original")] -> w14
      frame .."fire" {
      }
      frame "rainbow" {
      }
      frame "grey" {
      }
      frame "inverse grey" {
      }
      frame "ice" {
      }
      frame "original" {
      }
    }
    n26 = Reciprocal(x=w13) -> (1/x=w11:dbl)
    n27 = Bundle("Time steps"="Time steps", "Frequency bins"="Frequency bins") -> (w4:cluster{"Time steps":i32, "Frequency bins":i32})  [unwired: 1 in]
    n28 = Bundle("Type"="Type", "Length"="Length") -> (w19:cluster{"Type":u32, "Length":i32})  [unwired: 1 in]
    n29 = Unbundle By Name(w4) -> ("Time steps"=w18:i32, "Frequency bins"=w17:i32)
    n30 = call <vilib>:"STFT Spectrograms.vi"("window parameter"="Window parameter", "window info"=w19, "time-freq sampling info"=w4, "X"=w10) -> ("STFT Spectrogram {X}"=→"STFT Spectrogram":dbl[][])  [unwired: 2 in, 5 out]
    n31 = call <vilib>:"Auto Power Spectrum.vi"("dt"=w11, "Signal (V)"=w10) -> ("df"=w3:dbl, "Power Spectrum (V^2 rms)"=w7:dbl[])
    n32 = Multiply(x=w18, y=w11) -> (x*y=w16:dbl)
    n33 = Divide(x=w13, y=w17) -> (x/y=w15:dbl)
    n34 = Bundle By Name("Y"=w10, "dt"=w11) -> (→"Acquired time domain signal":waveform(dbl))  [unwired: 1 out]
    n35 = Array Size(array=w7) -> (size(s)=w9:i32)
    n36 = for {
      N: w9 -> [_]
      tunnel: [w29] -> w2 mode=indexing
      i -> [w29]
    }
    n37 = property on="STFT Spectrogram" class="IntGraph (strict)"("XScale.Multiplier"=w16, "YScale.Multiplier"=w15, "Color Table"=w14) -> ()  [unwired: 2 in, 2 out]
    n38 = Multiply(x=w3, y=w2) -> (x*y=w1:dbl[])
    n39 = Bundle("Power Spectrum (V^2 rms)"=w7, w1) -> (→"Power Spectrum":cluster{"Power Spectrum (V^2 rms)":dbl[], dbl[]})  [unwired: 1 out]
  }
